vi "MongoDB.FindAll.vi"(8 "error in (no error)":errorcluster, 11 "MongoDB.Collection in":refnum<class "MongoDB.Collection.lvclass">) -> (0 "error out":errorcluster, 2 "Result":string[](array[string]), 3 "MongoDB.Collection out":refnum<class "MongoDB.Collection.lvclass">)   [LabVIEW 2014, in "MongoDB.Collection.lvclass"]
uses:
  MongoDB.Collection.lvclass
  MongoDB.Collection.lvclass/MongoDB.Collection.ctl
  C:/Users/Richard/Documents/GitHub/mongo-labview-driver/CSharp/bin/MongoDB.Driver.Legacy.dll
  CSharp/bin/MongoDB.Driver.Legacy.dll
  C:/Users/Richard/Documents/GitHub/mongo-labview-driver/CSharp/bin/MongoDB.Bson.dll
  CSharp/bin/MongoDB.Bson.dll
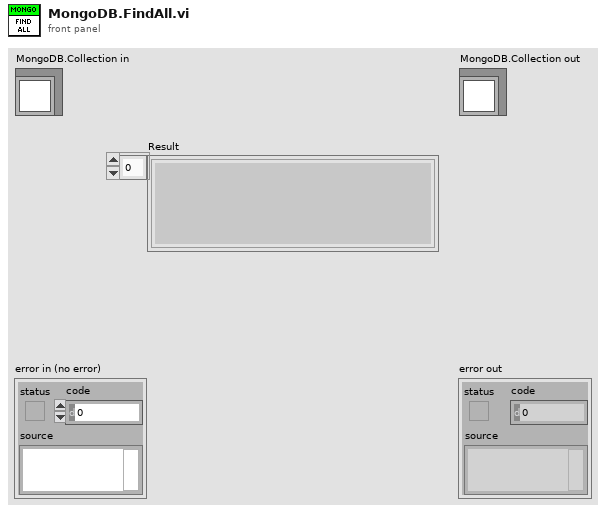
[diagram p1: front panel]
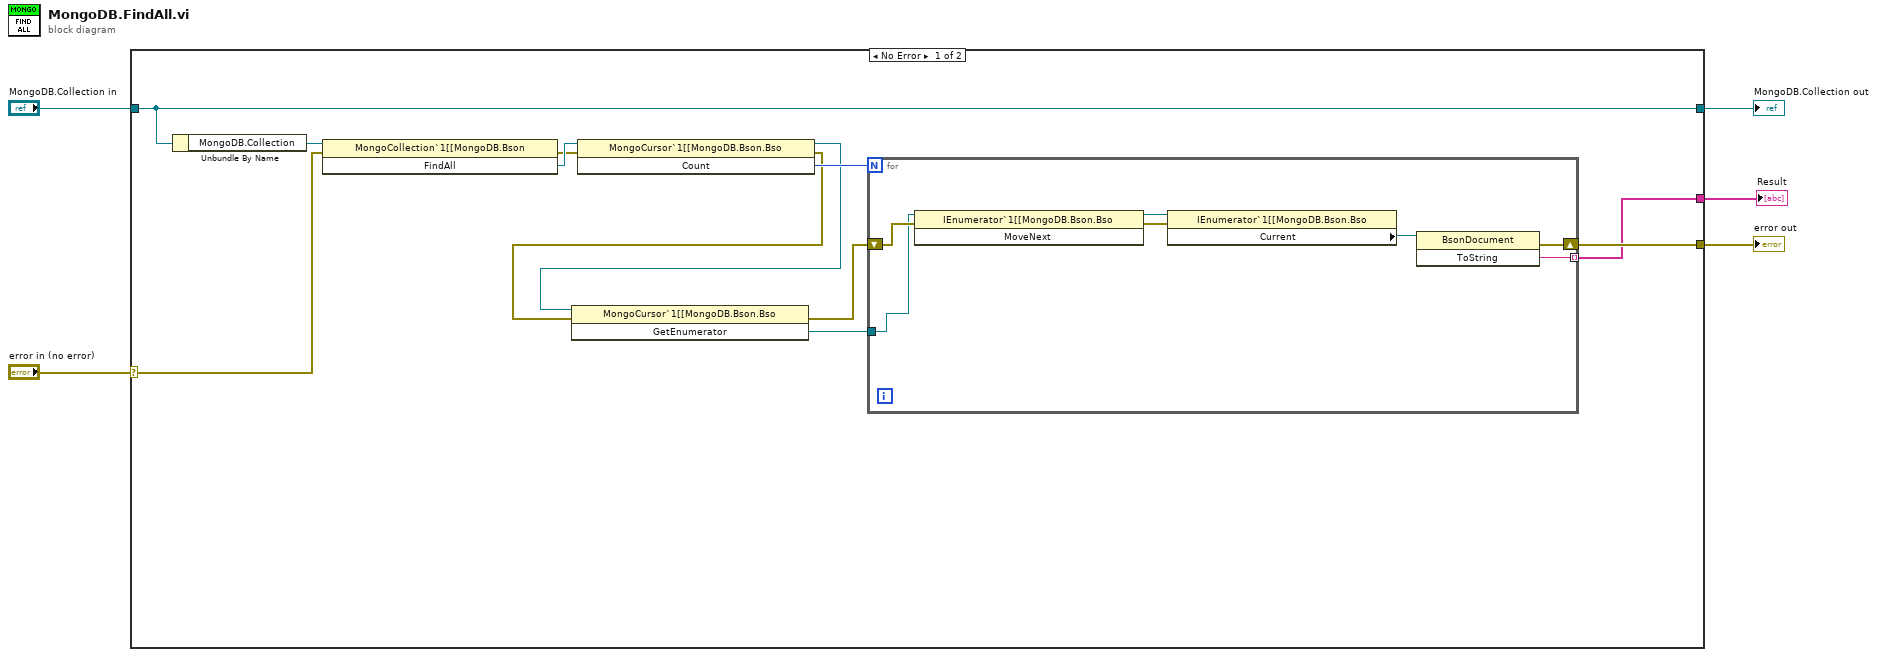
[diagram p0: block diagram]
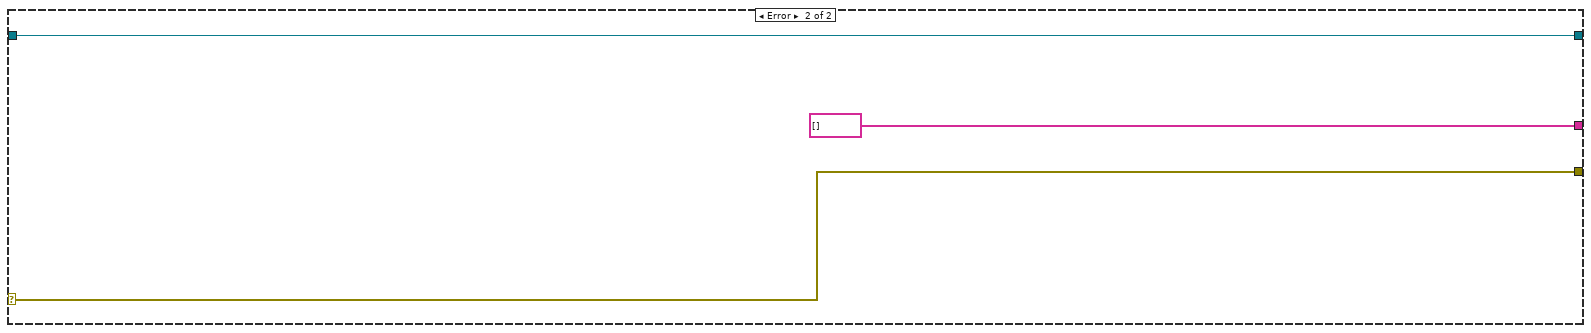
[diagram p2: hidden frame]
diagram:
  n1 = case shown="No Error" "error in (no error)" {
    selector: "error in (no error)" -> [w15 w27]
    tunnel: [w11 w27] -> w4
    tunnel: [w17 w26] -> w2
    tunnel: "MongoDB.Collection in" -> [w17 w26]
    tunnel: [w10 string[] []] -> w1
    frame No Error {
      n2 = Unbundle By Name(w17) -> ("MongoDB.Collection"=w16:refnum<k24>)
      n3 = invoke class="MongoCollection`1[[MongoDB.Bson" method="FindAll"(reference=w16, error in=w15) -> (error out=w12:errorcluster, "FindAll"=w14:refnum<k24>)  [unwired: 1 in, 1 out]
      n4 = invoke class="MongoCursor`1[[MongoDB.Bson.Bso" method="Count"(reference=w14, error in=w12) -> (reference out=w6:refnum<k24>, error out=w9:errorcluster, "Count"=w13:i64)  [unwired: 1 in]
      n5 = invoke class="MongoCursor`1[[MongoDB.Bson.Bso" method="GetEnumerator"(reference=w6, error in=w9) -> (error out=w8:errorcluster, "GetEnumerator"=w7:refnum<k24>)  [unwired: 1 in, 1 out]
      n6 = for {
        N: w13 -> [_]
        shift-right: [w18] -> w11
        shift-left: w8 -> [w22]
        tunnel: [w19] -> w10 mode=indexing
        tunnel: w7 -> [w21]
        n7 = invoke class="IEnumerator`1[[MongoDB.Bson.Bso" method="MoveNext"(reference=w21, error in=w22) -> (reference out=w24:refnum<k24>, error out=w23:errorcluster)  [unwired: 1 in, 1 out]
        n8 = property class="IEnumerator`1[[MongoDB.Bson.Bso"(reference=w24, error in=w23) -> ("Current"=w20:refnum<k24>)  [unwired: 2 out]
        n9 = invoke class="BsonDocument" method="ToString"(reference=w20) -> (error out=w18:errorcluster, "ToString"=w19:string)  [unwired: 2 in, 1 out]
      }
    }
    frame Error {
    }
  }
  "error out" <- w4
  "MongoDB.Collection out" <- w2
  "Result" <- w1
